vi "Command Settings.vi"() -> (5 "Command Stats":cluster{"Enum":T1, "U8":u8, "Payload":bool}[](array[cluster])=[{"Enum"=enum."Channel List", "U8"=0, "Payload"=TRUE}])   [LabVIEW 2021, in "ChnMngOOB_Tx.lvclass"]
uses:
  ChnMngOOB_Tx.lvclass
  Typedef/OOB Core Commands.ctl
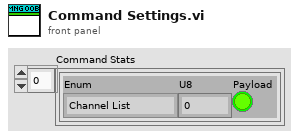
[diagram p1: front panel]
types:
  T1 = typedef "ChnMngOOB_Tx.lvclass/OOB Core Commands.ctl" = enum8{"Channel List", "New FIFO Pub"}
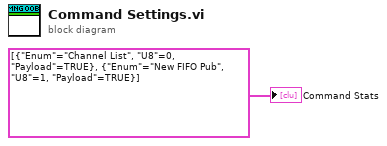
[diagram p0: block diagram]
diagram:
  "Command Stats" <- cluster{"Enum":T1, "U8":u8, "Payload":bool}[] [{"Enum"=enum."Channel List", "U8"=0, "Payload"=TRUE}, {"Enum"=enum."New FIFO Pub", "U8"=1, "Payload"=TRUE}]
